vi "HRR-MoveMultiplex.vi"(8 "error in (no error)":errorcluster, 10 "Array":u16[][](array[numeric]), 11 "Refnum in":refnum<k20>) -> (0 "error out":errorcluster, 3 "FPGA VI Reference Out":refnum<k20>)   [LabVIEW 2019]
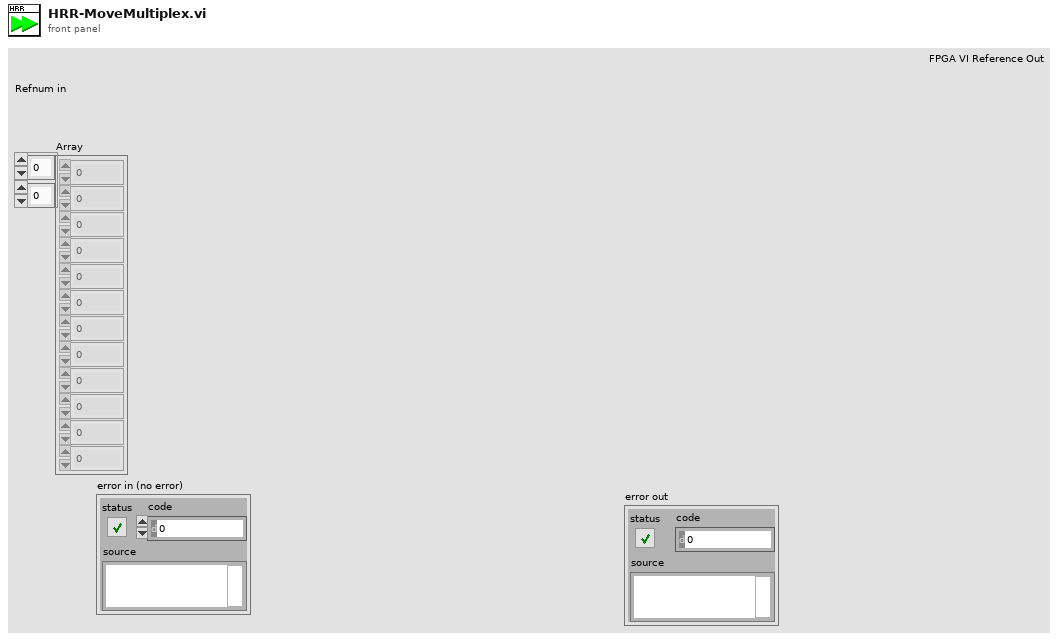
[diagram p1: front panel]
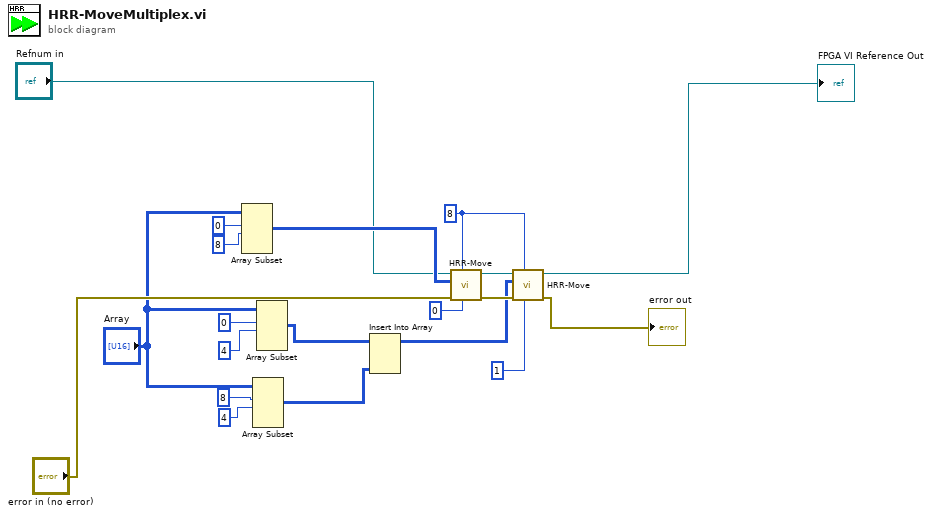
[diagram p0: block diagram]
diagram:
  w18 = 8 ("N° motores")
  n1 = Array Subset(array="Array", index (row)=0 ("index"), length (row)=8 ("length")) -> (w13:u16[][])  [unwired: 2 in]
  n2 = Array Subset(array="Array", index (row)=8 ("index"), length (row)=4 ("length")) -> (w9:u16[][])  [unwired: 2 in]
  n3 = Array Subset(array="Array", index (row)=0 ("index"), length (row)=4 ("length")) -> (w10:u16[][])  [unwired: 2 in]
  n4 = Insert Into Array(array=w10, new element=w9) -> (w8:u16[][])  [unwired: 2 in]
  n5 = call "HRR-Move.vi"("ID"=u8 0, "N° motores"=w18, "error in"="error in (no error)", "Pos, Vel"=w13, "FPGA VI Reference In"="Refnum in") -> ("error out"=w20:errorcluster, "FPGA VI Reference Out"=w19:refnum<k20>)  [unwired: 5 in]
  n6 = call "HRR-Move.vi"("ID"=u8 1, "N° motores"=w18, "error in"=w20, "Pos, Vel"=w8, "FPGA VI Reference In"=w19) -> ("error out"=→"error out":errorcluster, "FPGA VI Reference Out"=→"FPGA VI Reference Out":refnum<k20>)  [unwired: 5 in]
